vi "write to fifo.vi"(0 "p2p vst in":refnum<class "p2p vst.lvclass">, 11 "error in (no error)":errorcluster) -> (4 "p2p vst out":refnum<class "p2p vst.lvclass">, 6 "done write file":bool=TRUE, 8 "num of pulses sent to the FPGA":u32, 10 "room on fifo":bool=TRUE, 15 "error out":errorcluster)   [LabVIEW 2021, in "p2p vst.lvclass"]
uses:
  p2p vst.lvclass
  p2p vst.lvclass/p2p vst.ctl
  <vilib>/Utility/error.llb/Error Cluster From Error Code.vi
  <vilib>/rvi/errors/niLvFpgaAdjustHostInterfaceError.vi
  <vilib>/rvi/interface/nirviMethod/nirviMethod.xnode
  <vilib>/FPGAPlugInAG/Dynamic/niLvFpga_WriteFifo_Dynamic.vi
  <vilib>/rvi/errors/niLvFpgaMergeErrorWithErrorCode.vi
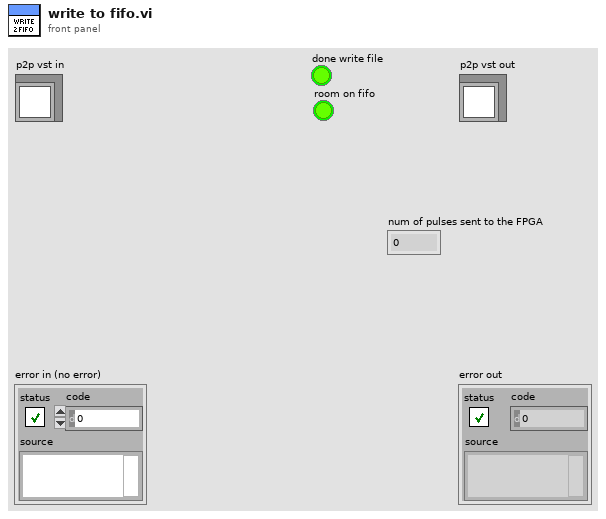
[diagram p1: front panel]
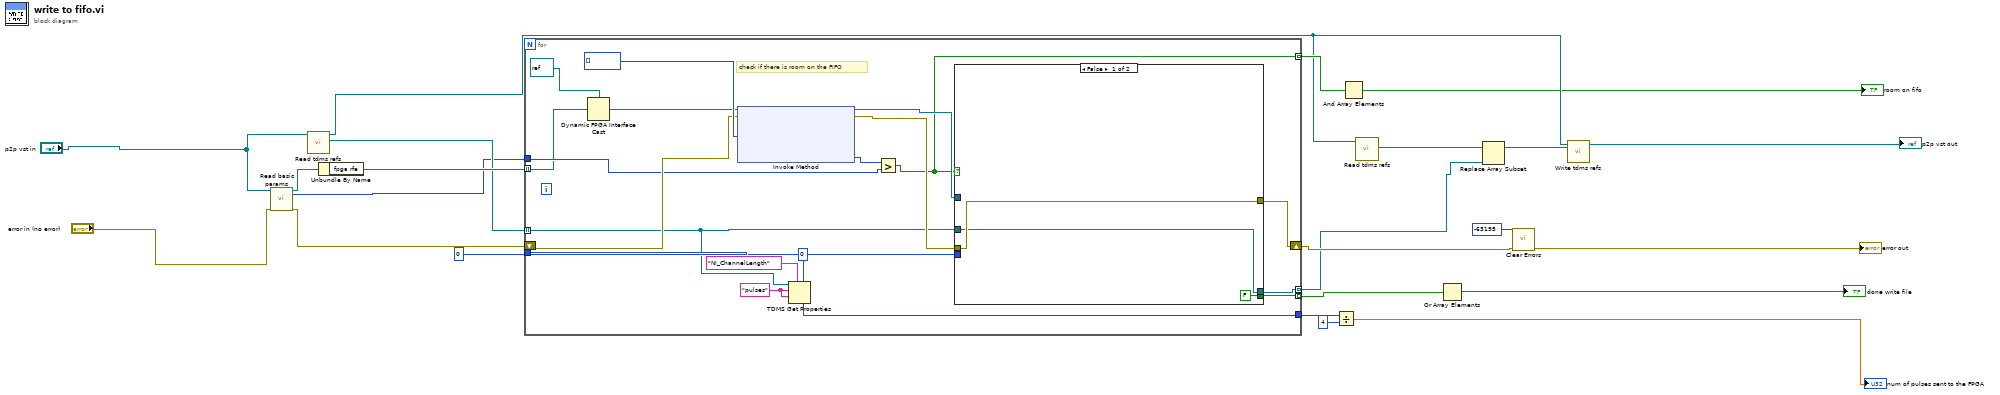
[diagram p0: block diagram]
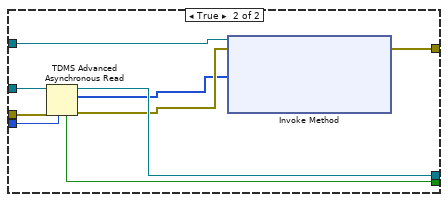
[diagram p2: hidden frame]
diagram:
  n1 = call-dynamic "Read basic params.vi"("device_type in"="p2p vst in", "error in (no error)"="error in (no error)") -> ("device_type out"=w11:refnum<class "p2p vst.lvclass">, "buffer size"=w12:u32, "error out"=w10:errorcluster)  [unwired: 12 in, 3 out]
  n2 = call-dynamic "Read tdms refs.vi"("device_type in"="p2p vst in") -> ("tdms refs"=w13:refnum<k34>[], "device_type out"=w8:refnum<class "p2p vst.lvclass">)  [unwired: 8 in, 1 out]
  n3 = Unbundle By Name(w11) -> ("fpga rfe"=w18:refnum<k20>[])
  n4 = for {
    tunnel: w13 -> [w25] mode=indexing
    tunnel: w18 -> [w31] mode=indexing
    tunnel: u64 0 ("type") -> [w42]
    tunnel: [w41] -> w19 mode=indexing
    tunnel: [w40] -> w14 mode=indexing
    shift-right: [w39] -> w16
    shift-left: w10 -> [w37]
    tunnel: [w24] -> w21
    tunnel: w12 -> [w36]
    tunnel: [w33] -> w15 mode=indexing
    w26 = "pulses" ("channel name")
    # "check if there is room on the FIFO"
    n5 = Dynamic FPGA Interface Cast(Session In=refnum<k20> refnum ("FPGA VI Reference Out"), Type=w31) -> (Session Out=w30:refnum<k20>)
    n6 = xnode "Invoke Method"("FPGA VI Reference In"=w30, "error in"=w37, "Data"=u64[] []) -> ("FPGA VI Reference Out"=w34:refnum<k20>, "error out"=w35:errorcluster, "Empty Elements Remaining"=w32:u32)  [unwired: 1 in]
    n7 = TDMS Get Properties(5:u64 0, 7:"NI_ChannelLength" ("property name"), 9:w26, 10:w26, 11:w25) -> (4:w24:u64)  [unwired: 1 in, 5 out]
    n8 = Greater?(x=w32, y=w36) -> (0:w33:bool)
    n9 = case shown="False" w33 {
      tunnel: w25 -> [w44 w54]
      tunnel: w42 -> [_ w53]
      tunnel: [FALSE ("read process finished?") w52] -> w41
      tunnel: [w44 w51] -> w40
      tunnel: [w45 w49] -> w39
      tunnel: w35 -> [w45 w47]
      tunnel: w34 -> [_ w46]
      frame False {
      }
      frame True {
        n10 = TDMS Advanced Asynchronous Read(6:w53, 8:w47, 11:w54) -> (0:w50:errorcluster, 2:w48:u64[], 3:w51:refnum<k34>, 4:w52:bool)
        n11 = xnode "Invoke Method"("FPGA VI Reference In"=w46, "error in"=w50, "Data"=w48) -> ("error out"=w49:errorcluster)  [unwired: 1 in, 2 out]
      }
    }
  }
  n12 = Divide(x=w21, y=4) -> (x/y=→"num of pulses sent to the FPGA":dbl)
  n13 = And Array Elements(Boolean array=w15) -> (logical AND=→"room on fifo":bool)
  n14 = call-dynamic "Read tdms refs.vi"("device_type in"=w8) -> ("tdms refs"=w9:refnum<k34>[])  [unwired: 8 in, 2 out]
  n15 = Or Array Elements(Boolean array=w19) -> (logical OR=→"done write file":bool)
  n16 = Replace Array Subset(array=w9, new element=w14) -> (w7:refnum<k34>[])  [unwired: 1 in]
  n17 = call <vilib>:"Clear Errors.vi"("error in (no error)"=w16, "specific error code to clear (0: all)"=-63195) -> ("error out"=→"error out":errorcluster)  [unwired: 4 in, 1 out]
  n18 = call-dynamic "Write tdms refs.vi"("tdms refs"=w7, "device_type in"=w8) -> ("device_type out"=→"p2p vst out":refnum<class "p2p vst.lvclass">)  [unwired: 8 in, 1 out]
